vi "PhotonPipelineResult_Pack.vi"(11 "PhotonPipelineResult_REF":T1) -> (3 "Packet_RawData":u8[](array[numeric]))   [LabVIEW 2019, in "PhotonVisionLib.lvlib"]
doc: "Convert a PipelineResult to a Packet array of bytes ready for writing to a Network Table variable.\n\nInputs:\n - PipelineResult -- PipelineResult cluster.\n\nOutputs:\n - Pacet_RawData -- Byte array containing the encoded PipelineResult."
uses:
  PhotonVisionLib.lvlib
  TypeDef/TargetCornerType.ctl
  TypeDef/PhotonTrackedTargetType.ctl
  TypeDef/PhotonPipelineResultType.ctl
  <vilib>/Rock Robotics/WPI/ThirdParty/JAS_Junk/TrajLib/TypeDef/TRANSLATION3D.ctl
  <vilib>/Rock Robotics/WPI/ThirdParty/JAS_Junk/TrajLib/Trajectory_Library.lvlib
  <vilib>/Rock Robotics/WPI/ThirdParty/JAS_Junk/TrajLib/TypeDef/QUATERNION.ctl
  <vilib>/Rock Robotics/WPI/ThirdParty/JAS_Junk/TrajLib/TypeDef/ROTATION3D.ctl
  <vilib>/Rock Robotics/WPI/ThirdParty/JAS_Junk/TrajLib/TypeDef/TRANSFORM3D.ctl
  TypeDef/PhotonPNPResultType.ctl
  TypeDef/PhotonMultiTargetPNPResultType.ctl
  Ref/PhotonPipelineResult_REF.ctl
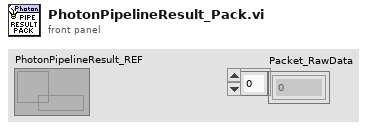
[diagram p1: front panel]
types:
  T1 = typedef "PhotonVisionLib.lvlib/PhotonPipelineResult_REF.ctl" = refnum<data-value>
  T2 = typedef "PhotonVisionLib.lvlib/PhotonMultiTargetPNPResultType.ctl" = cluster{"PhotonPNPResult":T3, "FiducialIDsUsed":i16[]}
  T3 = typedef "PhotonVisionLib.lvlib/PhotonPNPResultType.ctl" = cluster{"IsPresent":bool, "bestReprojErr":dbl, "altReprojErr":dbl, "ambiguity":dbl, "Best":T4, "Alt":T4}
  T4 = typedef "Trajectory_Library.lvlib/TRANSFORM3D.ctl" = cluster{"TRANSLATION3D":T5, "ROTATION3D":T6, "XF":bool}
  T5 = typedef "Trajectory_Library.lvlib/TRANSLATION3D.ctl" = cluster{"X":dbl, "Y":dbl, "Z":dbl}
  T6 = typedef "Trajectory_Library.lvlib/ROTATION3D.ctl" = cluster{"Q_quaternion":T7}
  T7 = typedef "Trajectory_Library.lvlib/QUATERNION.ctl" = cluster{"R":dbl, "V":dbl[]}
  T8 = typedef "PhotonVisionLib.lvlib/PhotonTrackedTargetType.ctl" = cluster{"Yaw":dbl, "Pitch":dbl, "Area":dbl, "Skew":dbl, "MinAreaRectCorners":T9[], "BestCameraToTarget":T4, "FiiducialId":i32, "AltCameraToTarget":T4, "PoseAmbiguity":dbl, "DetectedCorners":T9[]}
  T9 = typedef "PhotonVisionLib.lvlib/TargetCornerType.ctl" = cluster{"X":dbl, "Y":dbl}
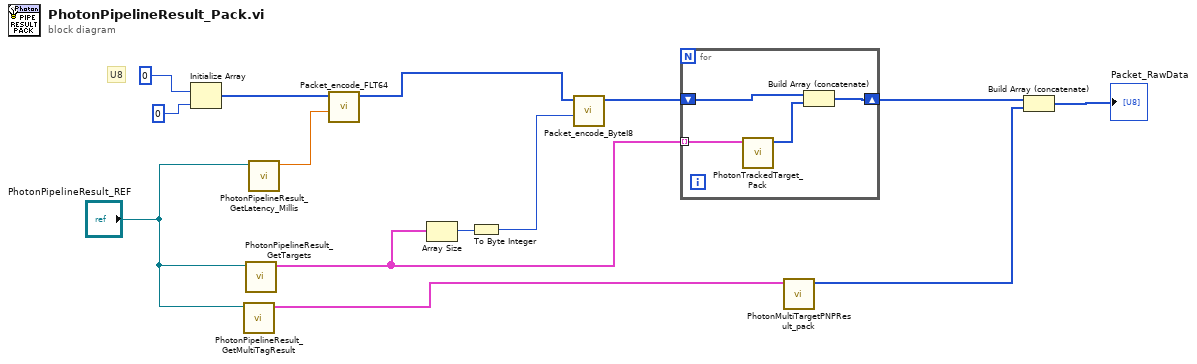
[diagram p0: block diagram]
diagram:
  # "U8"
  n1 = Initialize Array(u8 0 ("element"), 0 ("dimension size")) -> (w11:u8[])
  n2 = call "PhotonPipelineResult_GetMultiTagResult.vi"("PhotonPipelineResult_REF"="PhotonPipelineResult_REF") -> ("PhotonMultiTargetPNPResult"=w1:T2)  [unwired: 9 in, 1 out]
  n3 = call "PhotonPipelineResult_GetTargets.vi"("PhotonPipelineResult_REF"="PhotonPipelineResult_REF") -> ("Targets"=w2:T8[])  [unwired: 10 in]
  n4 = call "PhotonPipelineResult_GetLatency_Millis.vi"("PhotonPipelineResult_REF"="PhotonPipelineResult_REF") -> ("Latency_MilliSec"=w10:dbl)  [unwired: 9 in, 1 out]
  n5 = call "Packet_encode_FLT64.vi"("FLT64_Value"=w10, "RawData In"=w11) -> ("RawData Out"=w6:u8[])  [unwired: 9 in]
  n6 = Array Size(array=w2) -> (size(s)=w12:i32)
  n7 = To Byte Integer(number=w12) -> (8bit integer=w9:i8)
  n8 = call "Packet_encode_ByteI8.vi"("Int8_Value"=w9, "RawData In"=w6) -> ("RawData Out"=w8:u8[])  [unwired: 9 in]
  n9 = for {
    tunnel: w2 -> [w18] mode=indexing
    shift-right: [w15] -> w5
    shift-left: w8 -> [w17]
    n10 = call "PhotonTrackedTarget_Pack.vi"("TrackedTarget"=w18) -> ("RawData Out"=w16:u8[])  [unwired: 10 in]
    n11 = Build Array (concatenate)(w17, w16) -> (w15:u8[])
  }
  n12 = call "PhotonMultiTargetPNPResult_pack.vi"("MultiTargetPNP_Result"=w1) -> ("RawData Out"=w7:u8[])  [unwired: 10 in]
  n13 = Build Array (concatenate)(w5, w7) -> (→"Packet_RawData":u8[])
